vi "substates.vi"() -> (1 "Loop 2: Container Arm":T1, 2 "Loop 1: Lift":T1, 3 "Loop 0: Drive":T1)   [LabVIEW 2015]
uses:
  Type Defs/subStates.ctl
  <vilib>/Rock Robotics/Network Tables/NT Read Numeric Array.vi
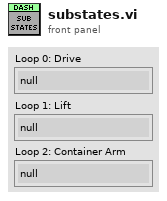
[diagram p1: front panel]
types:
  T1 = typedef "subStates.ctl" = enum16{"null", "wait", "driver control", "auto", "manual override", "hold position", "rotate", "test", "end"}
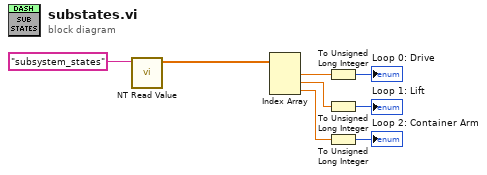
[diagram p0: block diagram]
diagram:
  n1 = call-poly <vilib>:"NT Read Value.vi"("Name"="subsystem_states") -> ("Numeric Array"=w7:dbl[])  [unwired: 9 in, 1 out]
  n2 = Index Array(array=w7) -> (element #1=w6:dbl, element #2=w3:dbl, element #3=w1:dbl)  [unwired: 3 in]
  n3 = To Unsigned Long Integer(number=w6) -> (unsigned 32bit integer=→"Loop 0: Drive":u32)
  n4 = To Unsigned Long Integer(number=w3) -> (unsigned 32bit integer=→"Loop 1: Lift":u32)
  n5 = To Unsigned Long Integer(number=w1) -> (unsigned 32bit integer=→"Loop 2: Container Arm":u32)
